vi "Read Stop Refnum.vi"(8 "error in (no error)":errorcluster, 11 "New Session in":refnum<class "New Session.lvclass">) -> (0 "error out":errorcluster, 2 "Stop Refnum":refnum<vi>, 3 "New Session out":refnum<class "New Session.lvclass">)   [LabVIEW 2016, in "New Session Class.lvlib" / "New Session.lvclass"]
uses:
  New Session.lvclass
  New Session.lvclass/New Session.ctl
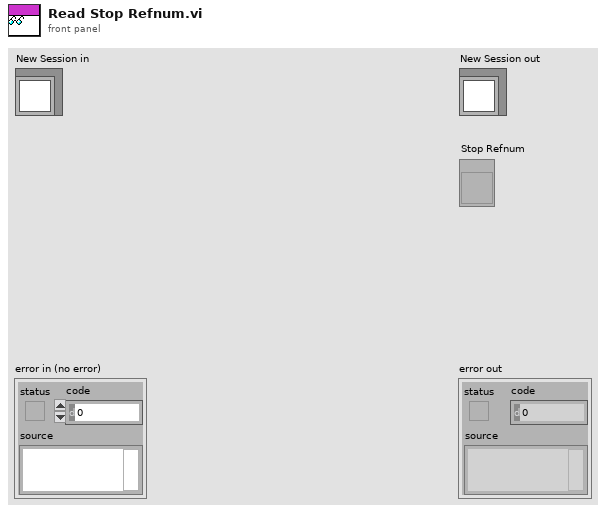
[diagram p1: front panel]
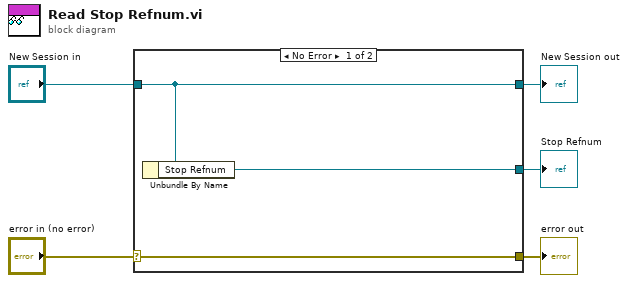
[diagram p0: block diagram]
diagram:
  n1 = case shown="No Error" "error in (no error)" {
    selector: "error in (no error)" -> [w8 w9]
    tunnel: [w8 w9] -> w4
    tunnel: [w7 w10] -> w2
    tunnel: "New Session in" -> [w7 w10]
    tunnel: [w6 _] -> w1
    frame No Error {
      n2 = Unbundle By Name(w7) -> ("Stop Refnum"=w6:refnum<vi>)
    }
    frame Error {
    }
  }
  "error out" <- w4
  "New Session out" <- w2
  "Stop Refnum" <- w1
